vi "Square root.vi"() -> ()   [LabVIEW 2014]
panel:
  out "Square Root":dbl
  in  "Number to Square Root":dbl=25.0 format="%#.0f"
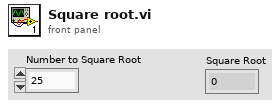
[diagram p1: front panel]
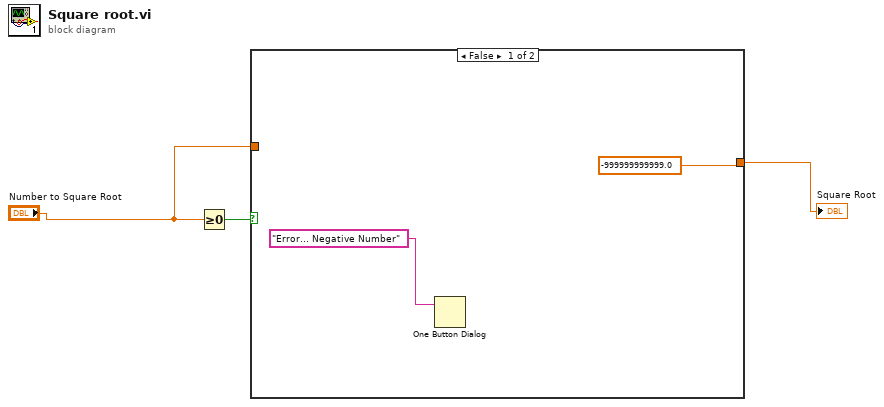
[diagram p0: block diagram]
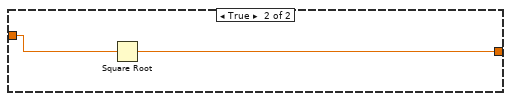
[diagram p2: hidden frame]
diagram:
  n1 = Greater Or Equal To 0?(x="Number to Square Root") -> (x >= 0?=w3:bool)
  n2 = case shown="False" w3 {
    tunnel: "Number to Square Root" -> [_ w7]
    tunnel: [-999999999999.0 ("Number to Square Root") w6] -> w1
    frame False {
      n3 = One Button Dialog(message="Error... Negative Number" ("button name (\"OK\")")) -> ()  [unwired: 1 in, 1 out]
    }
    frame True {
      n4 = Square Root(x=w7) -> (sqrt(x)=w6:dbl)
    }
  }
  "Square Root" <- w1
